vi "Commit.vi"(7 "New Branch (None)":string, 8 "error in (no error)":errorcluster, 9 "Message":string, 10 "Paths":string[](array[string]), 11 "Git Updater Module in":refnum<class "Git Updater Module.lvclass">) -> (0 "error out":errorcluster, 3 "Git Updater Module out":refnum<class "Git Updater Module.lvclass">)   [LabVIEW 2020, in "VolatusGUI.lvlib" / "Git Updater Module.lvclass"]
uses:
  Git Updater Module.lvclass
  Git Updater Module.lvclass/Git Updater Module.ctl
  <vilib>/Hampel Software Engineering/Git API/Git API/GIT-api.lvclass
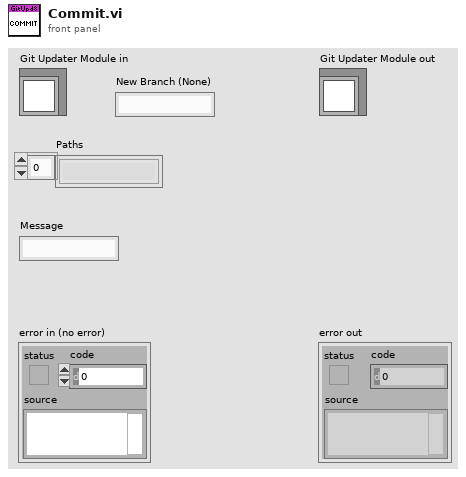
[diagram p1: front panel]
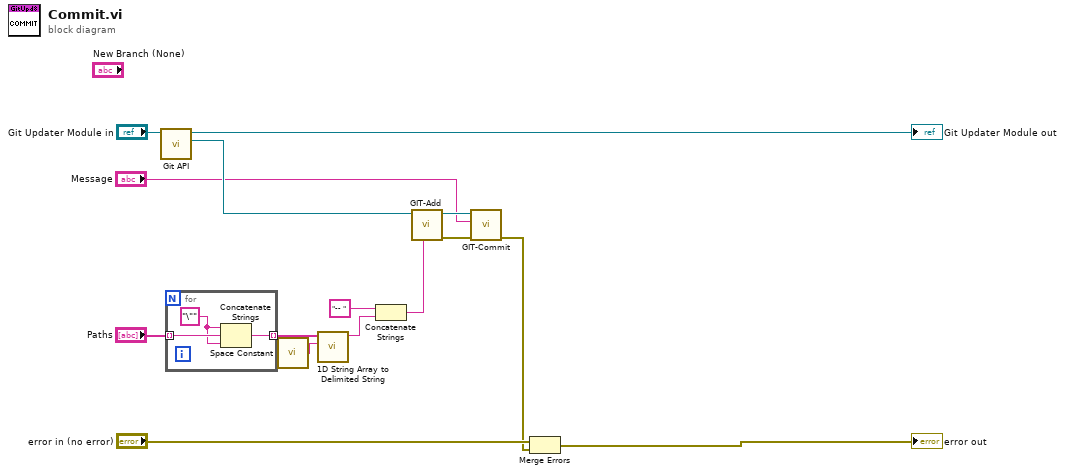
[diagram p0: block diagram]
diagram:
  n1 = call "Git API.vi"("Git Updater Module in"="Git Updater Module in") -> ("git-api"=w12:refnum<class "GIT-api.lvclass">, "Git Updater Module out"=→"Git Updater Module out":refnum<class "Git Updater Module.lvclass">)  [unwired: 8 in, 1 out]
  n2 = for {
    tunnel: "Paths" -> [w18] mode=indexing
    tunnel: [w16] -> w10 mode=indexing
    w17 = "\""
    n3 = Concatenate Strings(w17, w18, w17) -> (w16:string)
  }
  n4 = call <vilib>:"Space Constant.vi"() -> ("String"=w9:string)
  n5 = call <vilib>:"1D String Array to Delimited String.vi"("delimiter"=w9, "string array"=w10) -> ("delimited string"=w7:string)  [unwired: 9 in]
  n6 = Concatenate Strings("-- " ("string"), w7) -> (w6:string)
  n7 = call <vilib>:"GIT-Add.vi"("param"=w6, "git-api in"=w12) -> ("error out"=w5:errorcluster, "git-api out"=w4:refnum<class "GIT-api.lvclass">)  [unwired: 7 in, 1 out]
  n8 = call <vilib>:"GIT-Commit.vi"("error in"=w5, "msg"="Message", "Git-API in"=w4) -> ("error out"=w1:errorcluster)  [unwired: 7 in, 1 out]
  n9 = Merge Errors("error in (no error)", w1) -> (→"error out":errorcluster)
